vi "serialization-testing.vi"() -> ()   [LabVIEW 2018]
uses:
  Typedefs/key-value-type cluster.ctl
  demo/Component.lvclass
  demo/Implementations/Product-A.lvclass
  U:/modules/labview-orm/_Serializable Base Object/_ISerializable.lvclass
  U:/modules/labview-orm/demo/Product.lvclass
  Serializer/Serializer.lvclass
panel:
  out "Array":string[](array[string])
  out "status":u8
  in  "Boolean":bool
  in  "Numeric":i64
  out "Version":T1(array[cluster])
  out "Numeric read":i64
  out "owner read":string
  in  "owner":string
  out "serian-num read":dbl
  out "mayExplode_ read":bool
  in  "serian-num":dbl
  out "key-value-type":T2[](array[typedef])
  in  "id":i32
  out "id read":i32
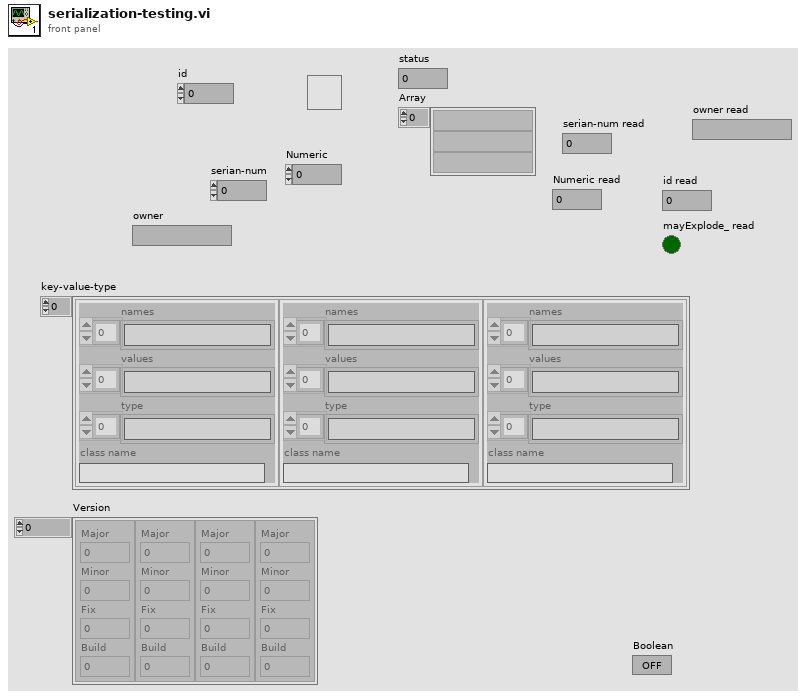
[diagram p1: front panel]
types:
  T1 = cluster{"Major":u16, "Minor":u16, "Fix":u16, "Build":u16}[]
  T2 = typedef "key-value-type cluster.ctl" = cluster{"names":string[], "values":string[], "type":string[], "class name":string}
  T3 = cluster{"Major":u16, "Minor":u16, "Fix":u16, "Build":u16}
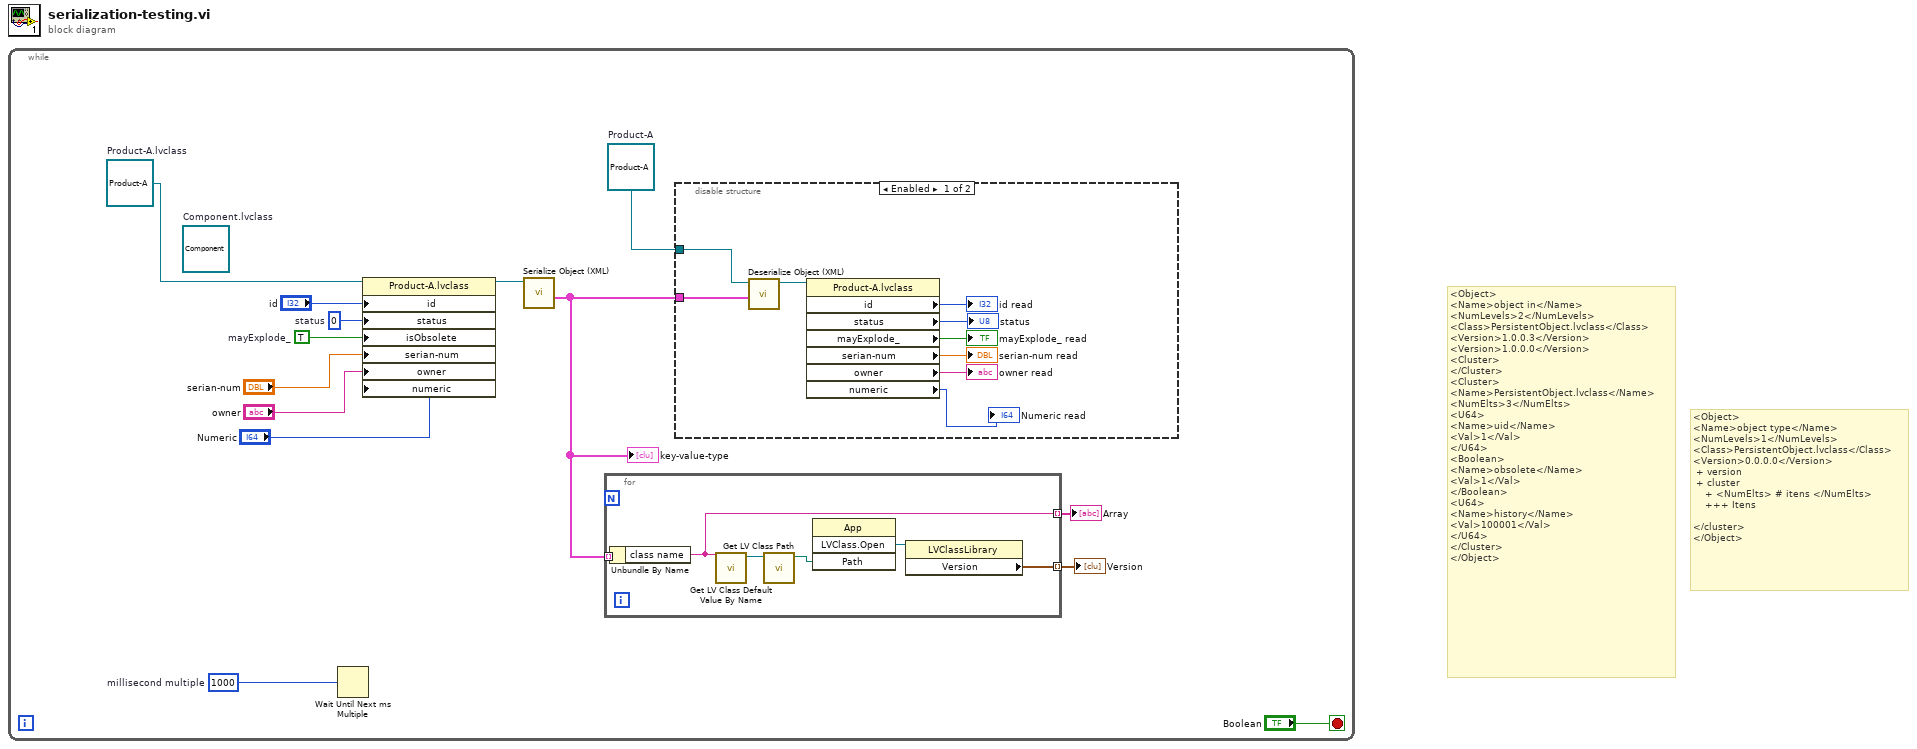
[diagram p0: block diagram]
diagram:
  # "<Object>\n<Name>object type</Name>\n<NumLevels>1</NumLevels>\n<Class>PersistentObject.lvclass</Class>\n<Version>0.0.0.0</Version>\n + version\n + cluster\n    + <NumElts> # itens </NumElts>\n    +++ Itens\n\n</cluster>\n</Object>"
  # "<Object>\n<Name>object in</Name>\n<NumLevels>2</NumLevels>\n<Class>PersistentObject.lvclass</Class>\n<Version>1.0.0.3</Version>\n<Version>1.0.0.0</Version>\n<Cluster>\n</Cluster>\n<Cluster>\n<Name>PersistentObject.lvclass</Name>\n<NumElts>3</NumElts>\n<U64>\n<Name>uid</Name>\n<Val>1</Val>\n</U64>\n<Boolean>\n<Name>obsolete</Name>\n<Val>1</Val>\n</Boolean>\n<U64>\n<Name>history</Name>\n<Val>100001</Val>\n</U64>\n</Cluster>\n</Object>"
  n1 = while {
    stop <- "Boolean" stop-if-true
    w3 = u8 0  # status
    w4 = refnum<class "Product-A.lvclass"> refnum  # Product-A.lvclass
    w6 = u32 1000  # millisecond multiple
    w9 = refnum<class "Product-A.lvclass"> refnum  # Product-A
    (unwired) refnum<class "Component.lvclass"> refnum  # Component.lvclass
    w12 = TRUE  # mayExplode_
    n2 = Wait Until Next ms Multiple(millisecond multiple=w6) -> ()  [unwired: 1 out]
    n3 = property class="Product-A.lvclass"(reference=w4, "id"="id", "status"=w3, "isObsolete"=w12, "serian-num"="serian-num", "owner"="owner", "numeric"="Numeric") -> (reference out=w14:refnum<class "Product-A.lvclass">)  [unwired: 1 in, 1 out]
    n4 = call "Serialize Object (XML).vi"("object in"=w14) -> ("key-value-type"=w1:T2[])  [unwired: 8 in, 2 out]
    "key-value-type" <- w1
    n5 = for {
      tunnel: w1 -> [w19] mode=indexing
      tunnel: [w16] -> w8 mode=indexing
      tunnel: [w15] -> w2 mode=indexing
      n6 = Unbundle By Name(w19) -> ("class name"=w15:string)
      n7 = call <vilib>:"Get LV Class Default Value By Name.vi"("class name"=w15) -> ("object"=w18:refnum<class>)  [unwired: 9 in, 1 out]
      n8 = call <vilib>:"Get LV Class Path.vi"("object"=w18) -> ("class path"=w17:path)  [unwired: 9 in, 1 out]
      n9 = invoke class="App" method="LVClass.Open"("Path"=w17) -> ("LVClass.Open"=w20:refnum<vi>)  [unwired: 3 in, 3 out]
      n10 = property class="LVClassLibrary"(reference=w20) -> ("Version"=w16:T3)  [unwired: 1 in, 2 out]
    }
    "Version" <- w8
    "Array" <- w2
    n11 = disable-structure shown="Enabled" {
      disable-tunnel: w9 -> [w29 _]
      disable-tunnel: w1 -> [w21 _]
      frame Enabled {
        n12 = call "Deserialize Object (XML).vi"("key-value-type in"=w21, "object type"=w29) -> ("object out"=w28:refnum<class "Product-A.lvclass">)  [unwired: 9 in]
        n13 = property class="Product-A.lvclass"(reference=w28) -> ("id"=→"id read":i32, "status"=→"status":u8, "mayExplode_"=→"mayExplode_ read":bool, "serian-num"=→"serian-num read":dbl, "owner"=→"owner read":string, "numeric"=→"Numeric read":i64)  [unwired: 1 in, 2 out]
      }
      frame Disabled {
      }
    }
  }
